vi "RobotStateWrite (SubVI).vi"(9 "time stamp":timestamp, 10 "string":string, 11 "Byte Stream File in":refnum<file>) -> ()   [LabVIEW 2013]
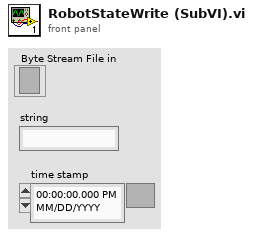
[diagram p1: front panel]
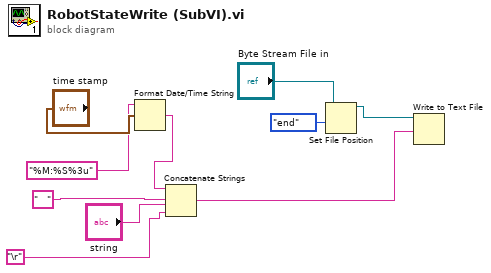
[diagram p0: block diagram]
diagram:
  n1 = Format Date/Time String(time format string (%c)="%M:%S%3u", seconds (now)="time stamp") -> (date/time string=w6:string)  [unwired: 1 in]
  n2 = Concatenate Strings(w6, "   ", "string", "\r") -> (w10:string)
  n3 = Set File Position(refnum="Byte Stream File in", from (0:start)=enum16{"start", "end", "current"}."end") -> (refnum out=w9:refnum<file>)  [unwired: 2 in, 1 out]
  n4 = Write to Text File(file (use dialog)=w9, text=w10) -> ()  [unwired: 2 in, 3 out]
